vi "Sine test with pre-offset.vi"(4 "DO Task":refnum<k21>="BlueSimple_DO", 5 "Sine parameters":T1={"Frequency"=0.5, "Degree displacement pk-pk"=90.0, "Cycles"=20} {"Degree displacement pk-pk" min=0.1 max=120.0; "Frequency" min=0.001 format="%#_4g"}) -> (1 "Return value":i16)   [LabVIEW 2010]
uses:
  Controls/Bits to Write.ctl
panel:
  out "sine offset size":string
  out "concatenated string":string
  out "x/y":dbl
  in  "precision (6)":i16=1
  out "String":string
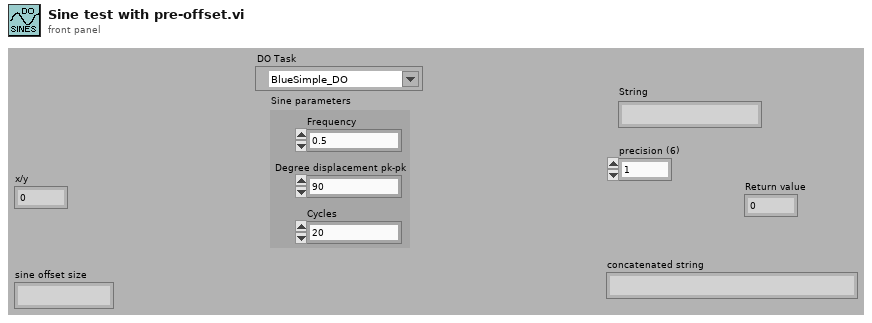
[diagram p1: front panel]
types:
  T1 = cluster{"Frequency":dbl, "Degree displacement pk-pk":dbl, "Cycles":i16}
  T2 = typedef "Bits to Write.ctl" = enum16{"LED 1 on", "LED 1 off", "LED 2 on", "LED 2 off", "LED 3 on", "LED 3 off", "LED 4 on", "LED 4 off", "All LEDs on", "All LEDs off", "In trial on", "In trial off", "Buzzer on", "Buzzer off", "Reward on", "Reward off", "Target number", "Trial type preQ on", "Trial type preQ off", "Error on", "Error off", "Trial number", "DBS on", "DBS off", "Sine on", "Sine off", "All Bits On", "All Bits Off", "Init", "Specify mask/pattern"}
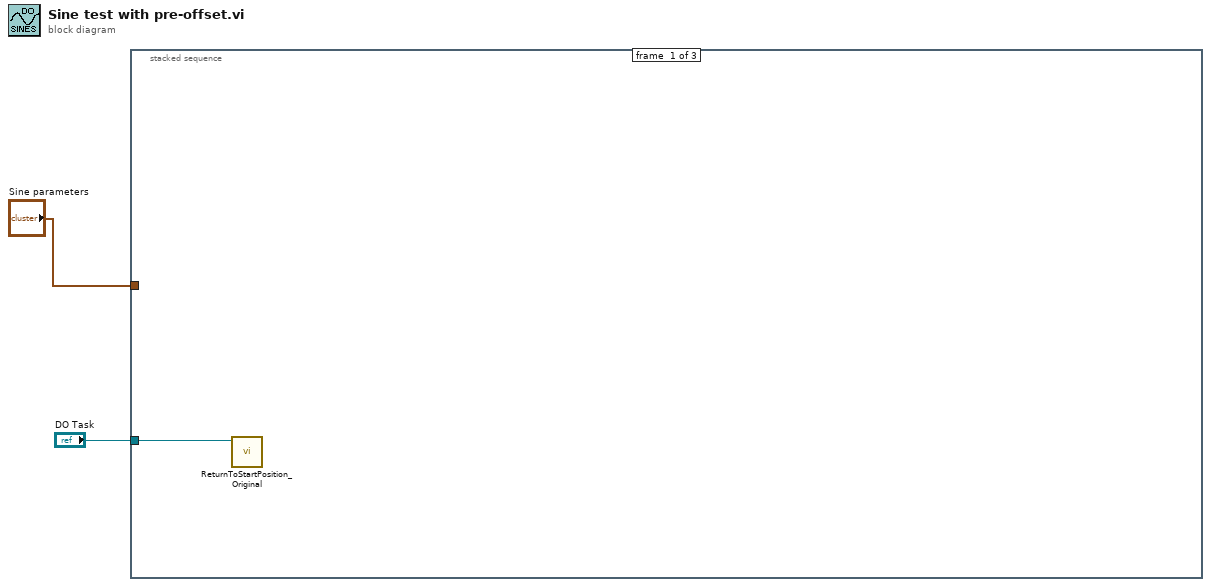
[diagram p0: block diagram]
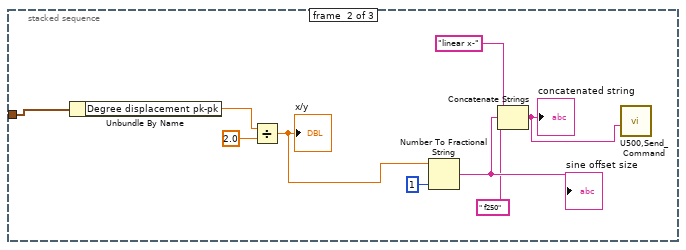
[diagram p2: hidden frame]
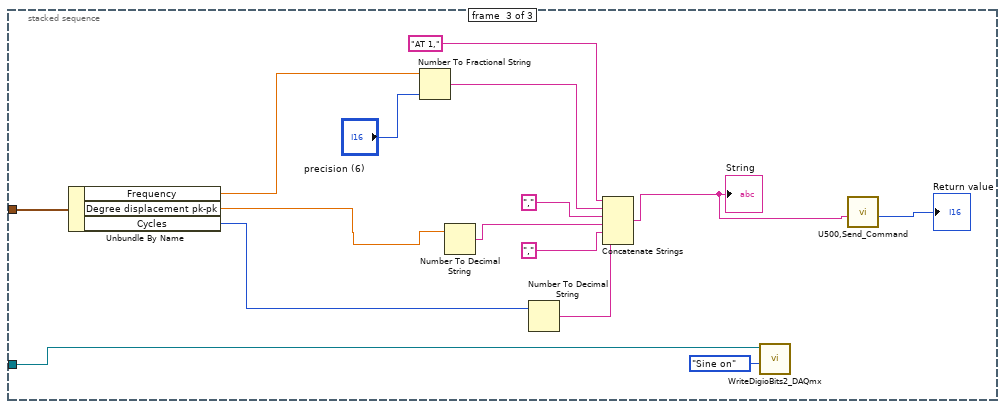
[diagram p3: hidden frame]
diagram:
  n1 = stacked-sequence {
    tunnel: "Sine parameters" -> [_ w5 w16]
    tunnel: "DO Task" -> [w3 _ w13]
    frame #0 {
      n2 = call "ReturnToStartPosition_Original.vi"("DO Task"=w3) -> ()  [unwired: 9 in]
    }
    frame #1 {
      n3 = Unbundle By Name(w5) -> ("Degree displacement pk-pk"=w12:dbl)
      n4 = Divide(x=w12, y=2.0) -> (x/y=w4:dbl)
      "x/y" <- w4
      n5 = Number To Fractional String(number=w4, precision (6)=i16 1) -> (F-format string=w8:string)  [unwired: 2 in]
      "sine offset size" <- w8
      n6 = Concatenate Strings("linear x-" ("Command String"), w8, " f250" ("string")) -> (w6:string)
      "concatenated string" <- w6
      n7 = call "U500,Send_Command.vi"("Command String"=w6) -> ()  [unwired: 9 in, 2 out]
    }
    frame #2 {
      n8 = Unbundle By Name(w16) -> ("Frequency"=w18:dbl, "Degree displacement pk-pk"=w15:dbl, "Cycles"=w17:i16)
      n9 = Number To Fractional String(number=w18, precision (6)="precision (6)") -> (F-format string=w25:string)  [unwired: 2 in]
      n10 = Number To Decimal String(number=w15) -> (decimal integer string=w23:string)  [unwired: 1 in]
      n11 = Number To Decimal String(number=w17) -> (decimal integer string=w21:string)  [unwired: 1 in]
      n12 = Concatenate Strings("AT 1," ("F-format string"), w25, "," ("F-format string"), w23, "," ("F-format string"), w21) -> (w20:string)
      "String" <- w20
      n13 = call "WriteDigioBits2_DAQmx.vi"("Bits to write"=Bits_to_Write."Sine on", "DO Task"=w13) -> ()  [unwired: 9 in, 1 out]
      n14 = call "U500,Send_Command.vi"("Command String"=w20) -> ("Return Value"=→"Return value":i16)  [unwired: 9 in, 1 out]
    }
  }
